vi "PI-TF.vi"(5 "Ki":sgl, 7 "Kp":sgl, 10 "setpoint":sgl, 11 "y(k)":sgl format="%#_13g") -> (1 "u(k)":sgl)   [LabVIEW 2017]
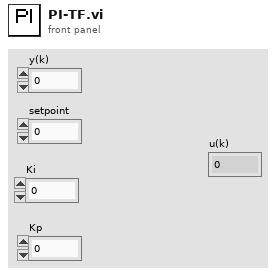
[diagram p1: front panel]
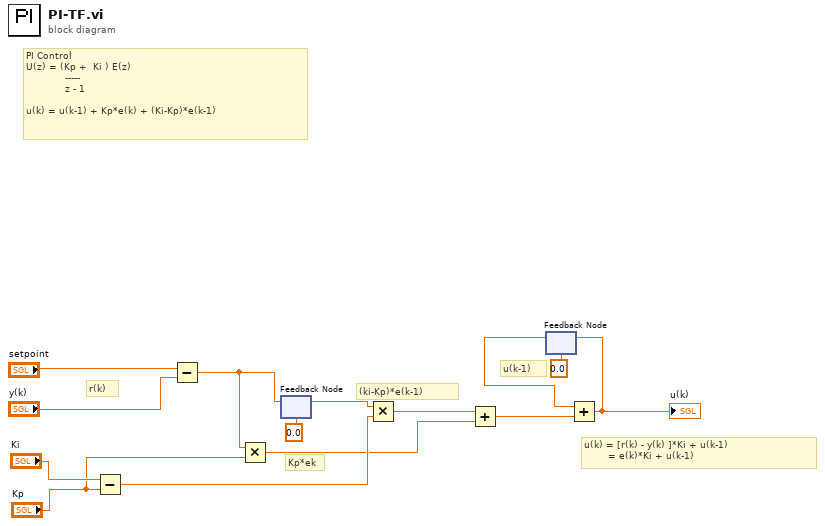
[diagram p0: block diagram]
diagram:
  # "Kp*ek"
  # "(ki-Kp)*e(k-1)"
  # "PI Control\nU(z) = (Kp +  Ki ) E(z)\n             -----\n             z - 1\n\nu(k) = u(k-1) + Kp*e(k) + (Ki-Kp)*e(k-1)"
  # "u(k) = [r(k) - y(k) ]*Ki + u(k-1)\n        = e(k)*Ki + u(k-1)"
  # "u(k-1)"
  # "r(k)"
  n1 = Subtract(x="Ki", y="Kp") -> (x-y=w9:sgl)
  n2 = Subtract(x="setpoint", y="y(k)") -> (x-y=w5:sgl)
  n3 = Multiply(x=w5, y="Kp") -> (x*y=w6:sgl)
  n4 = feedback-in #1(w5) -> ()
  n5 = feedback #1(sgl 0.0) -> (w10:sgl)
  n6 = Multiply(x=w10, y=w9) -> (x*y=w7:sgl)
  n7 = Add(x=w7, y=w6) -> (x+y=w4:sgl)
  n8 = feedback #2(sgl 0.0) -> (w1:sgl)
  n9 = Add(x=w1, y=w4) -> (x+y=w2:sgl)
  "u(k)" <- w2
  n10 = feedback-in #2(w2) -> ()
